vi "prime or non prime.vi"() -> ()   [LabVIEW 2012]
panel:
  out "String":string
  in  "Numeric":dbl
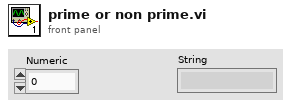
[diagram p1: front panel]
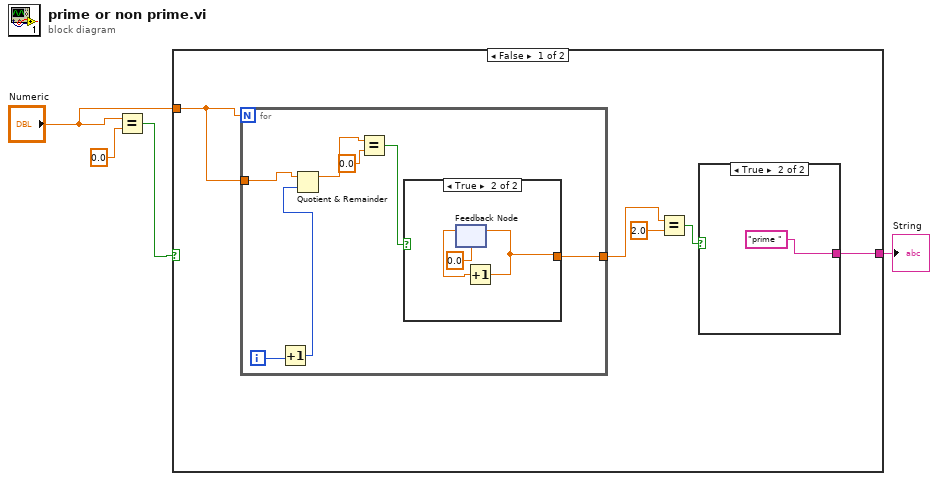
[diagram p0: block diagram]
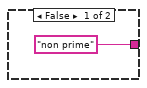
[diagram p2: hidden frame]
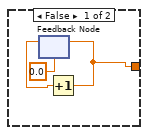
[diagram p3: hidden frame]
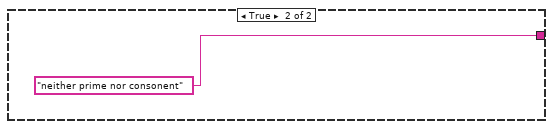
[diagram p4: hidden frame]
diagram:
  n1 = Equal?(x="Numeric", y=0.0) -> (x = y?=w3:bool)
  n2 = case shown="False" w3 {
    tunnel: "Numeric" -> [w9 _]
    tunnel: [w5 "neither prime nor consonent"] -> w1
    frame False {
      n3 = for {
        N: w9 -> [_]
        tunnel: w9 -> [w18]
        tunnel: [w13] -> w6
        i -> [w17]
        n4 = Increment(x=w17) -> (x+1=w16:i32)
        n5 = Quotient & Remainder(x=w18, y=w16) -> (x-y*floor(x/y)=w15:dbl)  [unwired: 1 out]
        n6 = Equal?(x=w15, y=0.0) -> (x = y?=w12:bool)
        n7 = case shown="True" w12 {
          tunnel: [w19 w22] -> w13
          frame False {
            n8 = feedback #1(0.0) -> (w21:dbl)
            n9 = Increment(x=w21) -> (x+1=w19:dbl)
            n10 = feedback-in #1(w19) -> ()
          }
          frame True {
            n11 = feedback #2(0.0) -> (w24:dbl)
            n12 = Increment(x=w24) -> (x+1=w22:dbl)
            n13 = feedback-in #2(w22) -> ()
          }
        }
      }
      n14 = Equal?(x=w6, y=2.0) -> (x = y?=w7:bool)
      n15 = case shown="True" w7 {
        tunnel: ["non prime" "prime "] -> w5
        frame False {
        }
        frame True {
        }
      }
    }
    frame True {
    }
  }
  "String" <- w1
